vi "Configure Descriptor Tables.vi"(7 "Virtual Memory Unit in":refnum<class "Virtual Memory Unit.lvclass">, 8 "error in (no error)":errorcluster, 11 "Remote Terminal in":refnum<class "Remote Terminal.lvclass">) -> (0 "error out":errorcluster, 3 "Remote Terminal out":refnum<class "Remote Terminal.lvclass">, 5 "Virtual Memory Unit out":refnum<class "Virtual Memory Unit.lvclass">)   [LabVIEW 2020, in "BCI-1553 API.lvlib" / "Remote Terminal.lvclass"]
doc: "Sets up the descriptor tables being leveraged for the operation of this RT. Circular Type 1 buffering is always used. Mode Codes should always use SMCP."
uses:
  Remote Terminal.lvclass
  Dependencies/Virtual Memory Unit/Virtual Memory Unit.lvclass
  Remote Terminal.lvclass/Remote Terminal.ctl
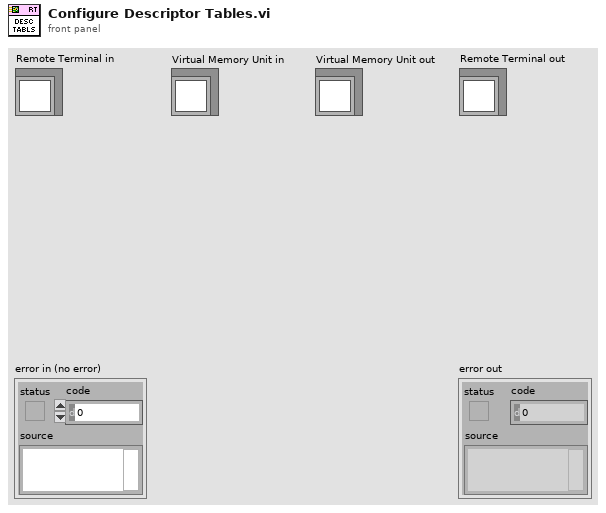
[diagram p1: front panel]
types:
  T1 = typedef "BCI-1553 API.lvlib/Remote Terminal.lvclass/RT CMD Config - Private.ctl" = cluster{"Command Type":T2, "SubAddress":T3, "Word Count\\Mode Code":T4, "Initial Data":u16[], "Data Fields":T5[]}
  T2 = typedef "BCI-1553 API.lvlib/Command Type.ctl" = enum16{"Transmit", "Receive"}
  T3 = typedef "BCI-1553 API.lvlib/Command SubAddress.ctl" = enum16{"Mode Code", "1", "2", "3", "4", "5", "6", "7", "8", "9", "10", "11", "12", "13", "14", "15", "16", "17", "18", "19", "20", "21", "22", "23", "24", "25", "26", "27", "28", "29", "30"}
  T4 = typedef "BCI-1553 API.lvlib/Command Word Count.ctl" = enum16{"1", "2", "3", "4", "5", "6", "7", "8", "9", "10", "11", "12", "13", "14", "15", "16", "17", "18", "19", "20", "21", "22", "23", "24", "25", "26", "27", "28", "29", "30", "31", "32"}
  T5 = typedef "BCI-1553 API.lvlib/Parameter Table Data.ctl" = cluster{"Parameter Name":string, "Base Word":u16, "Address":u16, "Value":u64, "Mask":u16[], "Scaling Info":T6}
  T6 = typedef "BCI-1553 API.lvlib/Scaling Information.ctl" = cluster{"Bit Offset":i32, "Bit Count":i32, "LSB Resolution":dbl, "2's Complement":bool, "Big Endian":bool, "Sign Bit":bool}
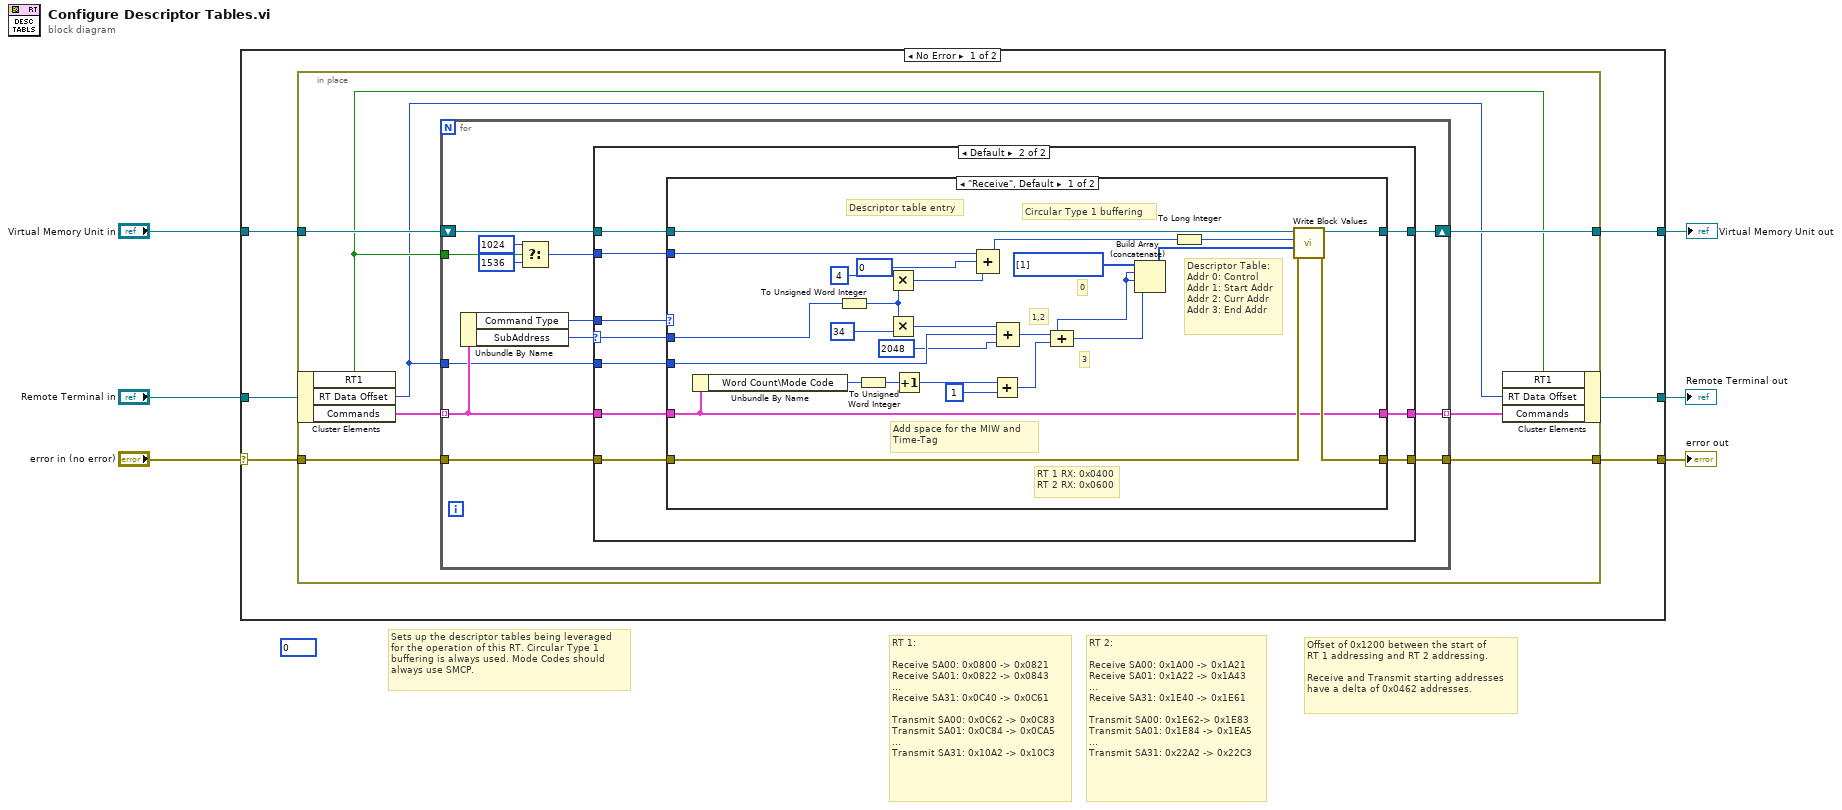
[diagram p0: block diagram]
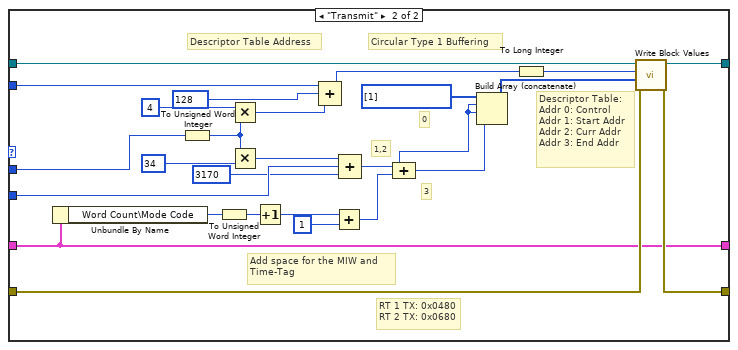
[diagram p3: hidden frame]
diagram:
  (unwired) u16 0 ("Address")
  # "Offset of 0x1200 between the start of\nRT 1 addressing and RT 2 addressing.\n\nReceive and Transmit starting addresses\nhave a delta of 0x0462 addresses."
  # "RT 2:\n\nReceive SA00: 0x1A00 -> 0x1A21\nReceive SA01: 0x1A22 -> 0x1A43\n...\nReceive SA31: 0x1E40 -> 0x1E61\n\nTransmit SA00: 0x1E62-> 0x1E83\nTransmit SA01: 0x1E84 -> 0x1EA5\n...\nTransmit SA31: 0x22A2 -> 0x22C3"
  # "RT 1:\n\nReceive SA00: 0x0800 -> 0x0821\nReceive SA01: 0x0822 -> 0x0843\n...\nReceive SA31: 0x0C40 -> 0x0C61\n\nTransmit SA00: 0x0C62 -> 0x0C83\nTransmit SA01: 0x0C84 -> 0x0CA5\n...\nTransmit SA31: 0x10A2 -> 0x10C3"
  # "Sets up the descriptor tables being leveraged\nfor the operation of this RT. Circular Type 1\nbuffering is always used. Mode Codes should\nalways use SMCP."
  n1 = case shown="No Error" "error in (no error)" {
    selector: "error in (no error)" -> [w10 w101]
    tunnel: [w9 w101] -> w5
    tunnel: [w7 w100] -> w3
    tunnel: "Remote Terminal in" -> [w12 w100]
    tunnel: "Virtual Memory Unit in" -> [w11 w99]
    tunnel: [w8 w99] -> w1
    frame No Error {
      n2 = in-place {
        in-place-border: w11 -> [w17]
        in-place-border: w10 -> [w19]
        in-place-border: [w20] -> w9
        in-place-border: [w16] -> w8
        n3 = in-place-cluster #1(w12) -> ("RT1"=w14:bool, "RT Data Offset"=w13:u16, "Commands"=w18:T1[])
        n4 = for {
          tunnel: [w29] -> w20
          tunnel: w19 -> [w33]
          tunnel: w18 -> [w27] mode=indexing
          shift-right: [w28] -> w16
          shift-left: w17 -> [w31]
          tunnel: [w30] -> w15 mode=indexing
          tunnel: w14 -> [w26]
          tunnel: w13 -> [w22]
          n5 = Unbundle By Name(w27) -> ("Command Type"=w32:T2, "SubAddress"=w21:T3)
          n6 = Select(t=u16 1024 ("Address"), s=w26, f=u16 1536 ("Address")) -> (s? t:f=w23:u16)
          n7 = case shown="Default" w21 {
            selector: w21 -> [_ w37]
            tunnel: w33 -> [w34 w46]
            tunnel: w32 -> [_ w45]
            tunnel: w31 -> [w35 w44]
            tunnel: [w36 w43] -> w30
            tunnel: [w34 w42] -> w29
            tunnel: [w35 w41] -> w28
            tunnel: w27 -> [w36 w40]
            tunnel: w23 -> [_ w39]
            tunnel: w22 -> [_ w38]
            frame "Mode Code" {
              # "Doesn't need any configuration."
              # "Uses SMCP.\nUses descriptor table words directly\nfor MIW, TimeTag, and Data Word\nstorage."
            }
            frame Default {
              n8 = case shown="\"Receive\", Default" w45 {
                tunnel: w46 -> [w64 w90]
                tunnel: w40 -> [w56 w82]
                tunnel: w44 -> [w70 w96]
                tunnel: [w56 w82] -> w43
                tunnel: [w63 w89] -> w42
                tunnel: [w69 w95] -> w41
                tunnel: w39 -> [w71 w97]
                tunnel: w38 -> [w60 w86]
                tunnel: w37 -> [w48 w74]
                frame "Receive", Default {
                  # "Descriptor table entry"
                  # "Circular Type 1 buffering"
                  # "3"
                  # "1,2"
                  # "0"
                  # "Add space for the MIW and\nTime-Tag"
                  # "Descriptor Table:\nAddr 0: Control\nAddr 1: Start Addr\nAddr 2: Curr Addr\nAddr 3: End Addr"
                  # "RT 1 RX: 0x0400\nRT 2 RX: 0x0600"
                  n9 = Unbundle By Name(w56) -> ("Word Count\\Mode Code"=w54:T4)
                  n10 = To Unsigned Word Integer(number=w48) -> (unsigned 16bit integer=w47:u16)
                  n11 = To Unsigned Word Integer(number=w54) -> (unsigned 16bit integer=w50:u16)
                  n12 = Multiply(x=u16 4 ("y"), y=w47) -> (x*y=w65:u16)
                  n13 = Multiply(x=w47, y=u16 34 ("Address")) -> (x*y=w61:u16)
                  n14 = Increment(x=w50) -> (x+1=w49:u16)
                  n15 = Compound Arithmetic op=ADD(w71, u16 0 ("Address"), w65) -> (w68:u16)
                  n16 = Add(x=w49, y=u16 1) -> (x+y=w55:u16)
                  n17 = Compound Arithmetic op=ADD(w61, w60, u16 2048 ("Address")) -> (w51:u16)
                  n18 = Compound Arithmetic op=ADD(w51, w55) -> (w52:u16)
                  n19 = Build Array (concatenate)(u16[] [1] ("Address"), w51, w51, w52) -> (w57:u16[])
                  n20 = To Long Integer(number=w68) -> (32bit integer=w67:i32)
                  n21 = call "Write Block Values.vi"("error in (no error)"=w64, "Write Block"=w57, "Start Index"=w67, "Virtual Memory Unit in"=w70) -> ("error out"=w63:errorcluster, "Virtual Memory Unit out"=w69:refnum<class "Virtual Memory Unit.lvclass">)  [unwired: 6 in]
                }
                frame "Transmit" {
                  # "Circular Type 1 Buffering"
                  # "Descriptor Table Address"
                  # "3"
                  # "1,2"
                  # "0"
                  # "Add space for the MIW and\nTime-Tag"
                  # "Descriptor Table:\nAddr 0: Control\nAddr 1: Start Addr\nAddr 2: Curr Addr\nAddr 3: End Addr"
                  # "RT 1 TX: 0x0480\nRT 2 TX: 0x0680"
                  n22 = Unbundle By Name(w82) -> ("Word Count\\Mode Code"=w80:T4)
                  n23 = To Unsigned Word Integer(number=w74) -> (unsigned 16bit integer=w73:u16)
                  n24 = To Unsigned Word Integer(number=w80) -> (unsigned 16bit integer=w76:u16)
                  n25 = Multiply(x=u16 4 ("y"), y=w73) -> (x*y=w91:u16)
                  n26 = Multiply(x=w73, y=u16 34 ("Address")) -> (x*y=w87:u16)
                  n27 = Increment(x=w76) -> (x+1=w75:u16)
                  n28 = Compound Arithmetic op=ADD(w97, u16 128 ("Address"), w91) -> (w94:u16)
                  n29 = Add(x=w75, y=u16 1) -> (x+y=w81:u16)
                  n30 = Compound Arithmetic op=ADD(w87, w86, u16 3170 ("Address")) -> (w77:u16)
                  n31 = Compound Arithmetic op=ADD(w77, w81) -> (w78:u16)
                  n32 = Build Array (concatenate)(u16[] [1] ("Address"), w77, w77, w78) -> (w83:u16[])
                  n33 = To Long Integer(number=w94) -> (32bit integer=w93:i32)
                  n34 = call "Write Block Values.vi"("error in (no error)"=w90, "Write Block"=w83, "Start Index"=w93, "Virtual Memory Unit in"=w96) -> ("error out"=w89:errorcluster, "Virtual Memory Unit out"=w95:refnum<class "Virtual Memory Unit.lvclass">)  [unwired: 6 in]
                }
              }
            }
          }
        }
        n35 = in-place-cluster #1("RT1"=w14, "RT Data Offset"=w13, "Commands"=w15) -> (w7:refnum<class "Remote Terminal.lvclass">)
      }
    }
    frame Error {
    }
  }
  "error out" <- w5
  "Remote Terminal out" <- w3
  "Virtual Memory Unit out" <- w1
